vi "ElmoVelInScale.vi"(1 "Elmo eCAT vel (ticks/s)":i32) -> (0 "Elmo vel (rad/s)":dbl)   [LabVIEW 2018]
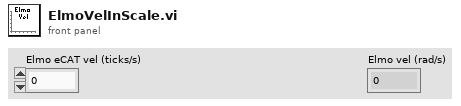
[diagram p1: front panel]
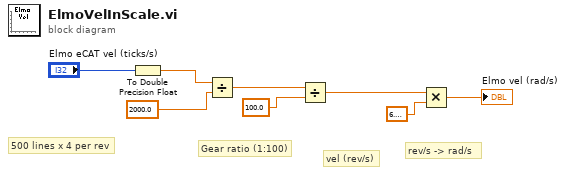
[diagram p0: block diagram]
diagram:
  # "rev/s -> rad/s"
  # "vel (rev/s)"
  # "500 lines x 4 per rev"
  # "Gear ratio (1:100)"
  n1 = To Double Precision Float(number="Elmo eCAT vel (ticks/s)") -> (double precision float=w8:dbl)
  n2 = Divide(x=w8, y=2000.0) -> (x/y=w6:dbl)
  n3 = Divide(x=w6, y=100.0) -> (x/y=w3:dbl)
  n4 = Multiply(x=w3, y=6.283185307179586) -> (x*y=→"Elmo vel (rad/s)":dbl)
